vi "sort_and_index2.vi"(2 "Ascending?":bool, 3 "Presorted Array":dbl[](array[numeric])=[4.0, 6.0, 3.0, 2.0] format="%.2f") -> (0 "Index":i32[](array[numeric])=[3, 2, 0, 1], 1 "Sorted Array":dbl[](array[numeric])=[2.0, 3.0, 4.0, 6.0] format="%.2f")   [LabVIEW 2017]
doc: "This example VI sorts a 1D array and provides an index matrix\n\nThis VI uses the Index and Bundle Cluster Array function to bundle an array and a set of indices. Then, this VI uses the Sort 1D Array function and a For Loop to generate a sorted array.\n\nThe following example demonstrates the sorting capabilities of this VI.\nunsorted array A=[5 4 5 3 1 2]\nsorted array B = [1 2 3 4 5 5]\nindex of A after sorted = [4 5 3 1 0 2]"
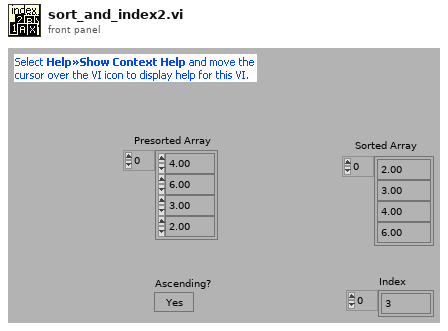
[diagram p1: front panel]
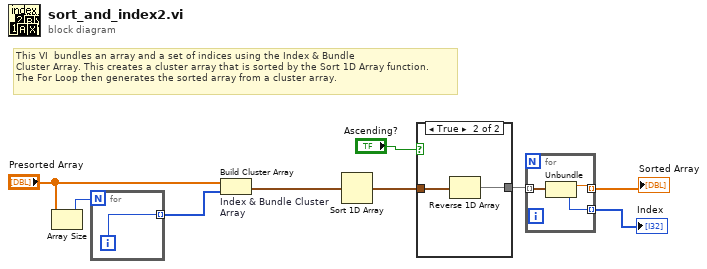
[diagram p0: block diagram]
diagram:
  # "This VI  bundles an array and a set of indices using the Index & Bundle\nCluster Array. This creates a cluster array that is sorted by the Sort 1D Array function.\nThe For Loop then generates the sorted array from a cluster array."
  n1 = Array Size(array="Presorted Array") -> (size(s)=w7:i32)
  n2 = for {
    N: w7 -> [_]
    tunnel: [w10] -> w6 mode=indexing
    i -> [w10]
  }
  n3 = Build Cluster Array "Index & Bundle Cluster Array"("Presorted Array", w6) -> (w9:cluster{dbl, i32}[])
  n4 = Sort 1D Array(array=w9) -> (sorted array=w3:cluster{dbl, i32}[])
  n5 = case shown="True" "Ascending?" {
    tunnel: w3 -> [w11 w13]
    tunnel: [w11 w12] -> w2
    frame False {
    }
    frame True {
      n6 = Reverse 1D Array(array=w13) -> (reversed array=w12:cluster{dbl, i32}[])
    }
  }
  n7 = for {
    tunnel: w2 -> [w16] mode=indexing
    tunnel: [w15] -> w5 mode=indexing
    tunnel: [w14] -> w4 mode=indexing
    n8 = Unbundle(w16) -> (w15:dbl, w14:i32)
  }
  "Sorted Array" <- w5
  "Index" <- w4
